vi "Parse N Packets.vi"(9 "Num Packets":i32, 10 "Capture Lengths":T1, 11 "data":string) -> (0 "destination addresses":string[](array[string]), 1 "source addresses":string[](array[string]), 2 "ip headers":T2[](array[typedef]) {"options / padding" format="%02x"; "fragment offset" format="%04x"; "IHL" format="%02x"; "version" format="%01x"; "type of service" format="%02x"; "total length" format="%02x"; "identification" format="%04x"; "flags" format="%.0x"; "time to live" format="%02x"; "protocol" format="%02.0f"; "header checksum" format="%04x"; "source address" format="%08x"; "destination address" format="%08x"}, 3 "ethernet headers":T3[](array[typedef]) {"destination MAC address"."?" format="%02x"; "destination MAC address"."?" format="%02x"; "destination MAC address"."?" format="%02x"; "destination MAC address"."?" format="%02x"; "destination MAC address"."?" format="%02x"; "destination MAC address"."?" format="%02x"; "source MAC address"."?" format="%02x"; "source MAC address"."?" format="%02x"; "source MAC address"."?" format="%02x"; "source MAC address"."?" format="%02x"; "source MAC address"."?" format="%02x"; "source MAC address"."?" format="%02x"; "length / type" format="%04x"}, 4 "ip datas":string[](array[string]), 5 "ip packets":bool[](array[boolean]))   [LabVIEW 2025, in "Automotive Ethernet Bus Monitor UI.lvlib" / "lvwpcap.lvlib"]
doc: "This VI parses out the ethernet and IP header from each incoming packet. It does not parse out any TCP or UDP headers. See the block diagram for more information on adding this functionality."
uses:
  lvwpcap.lvlib
  types/control_packet_header_ethernet.ctl
  types/control_packet_header_ip.ctl
  types/Capture Legnths.ctl
panel:
  # "Select Help»Show Context Help and move the cursor over the VI icon to display help for this VI."
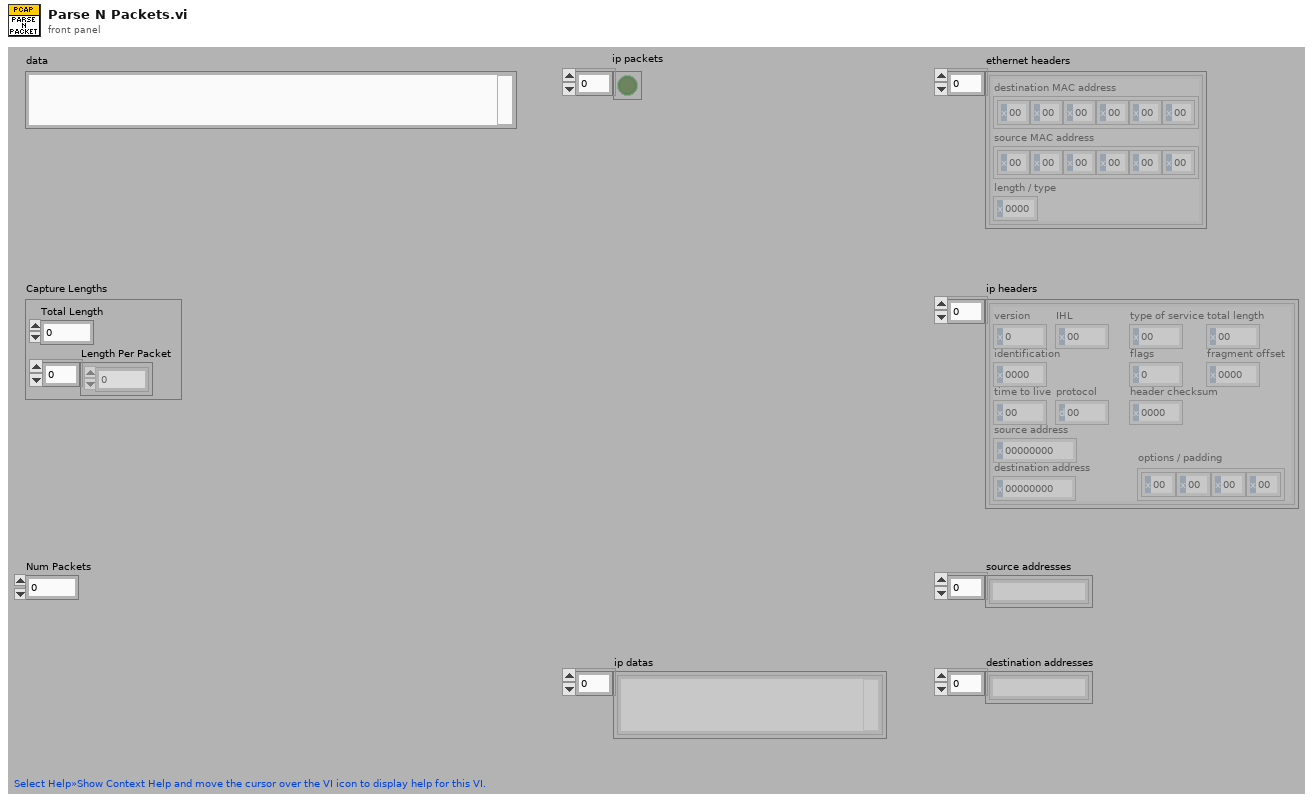
[diagram p1: front panel]
types:
  T1 = typedef "Automotive Ethernet Bus Monitor UI.lvlib/lvwpcap.lvlib/Capture Legnths.ctl" = cluster{"Total Length":u32, "Length Per Packet":u32[]}
  T2 = typedef "Automotive Ethernet Bus Monitor UI.lvlib/lvwpcap.lvlib/control_packet_header_ip.ctl" = cluster{"version":u8, "IHL":u8, "type of service":u8, "total length":u16, "identification":u16, "flags":u16, "fragment offset":u16, "time to live":u8, "protocol":u8, "header checksum":u16, "source address":u32, "destination address":u32, "options / padding":u8[]}
  T3 = typedef "Automotive Ethernet Bus Monitor UI.lvlib/lvwpcap.lvlib/control_packet_header_ethernet.ctl" = cluster{"destination MAC address":cluster{u8, u8, u8, u8, u8, u8}, "source MAC address":cluster{u8, u8, u8, u8, u8, u8}, "length / type":u16}
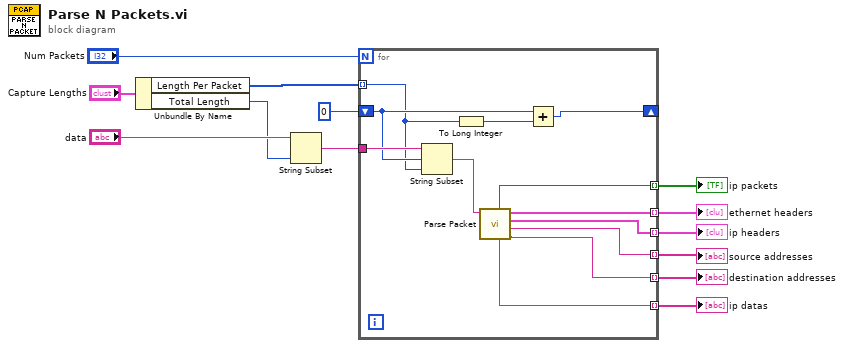
[diagram p0: block diagram]
diagram:
  n1 = Unbundle By Name("Capture Lengths") -> ("Length Per Packet"=w2:u32[], "Total Length"=w5:u32)
  n2 = String Subset(string="data", length (rest)=w5) -> (substring=w3:string)  [unwired: 1 in]
  n3 = for {
    N: "Num Packets" -> [_]
    tunnel: [w25] -> w13 mode=indexing
    tunnel: [w24] -> w12 mode=indexing
    tunnel: [w23] -> w11 mode=indexing
    tunnel: [w22] -> w10 mode=indexing
    tunnel: [w21] -> w9 mode=indexing
    tunnel: [w20] -> w7 mode=indexing
    tunnel: w3 -> [w19]
    tunnel: w2 -> [w17] mode=indexing
    shift-right: [w15] -> _
    shift-left: 0 ("offset (0)") -> [w18]
    n4 = String Subset(string=w19, offset (0)=w18, length (rest)=w17) -> (substring=w14:string)
    n5 = To Long Integer(number=w17) -> (32bit integer=w16:i32)
    n6 = call "Parse Packet.vi"("data"=w14) -> ("destination address"=w22:string, "source address"=w23:string, "ip header"=w24:T2, "ethernet header"=w25:T3, "ip data"=w21:string, "ip packet"=w20:bool)  [unwired: 5 in]
    n7 = Add(x=w18, y=w16) -> (x+y=w15:i32)
  }
  "ethernet headers" <- w13
  "ip datas" <- w9
  "source addresses" <- w11
  "destination addresses" <- w10
  "ip headers" <- w12
  "ip packets" <- w7
